vi "AB_Check_ConPane_For_Terminal_Type.vi"(8 "error in (no error)":errorcluster, 10 "Type Enum":T1, 11 "VI Path":path) -> (0 "error out":errorcluster, 3 "type found":bool)   [LabVIEW 2020]
uses:
  <vilib>/Utility/VariantDataType/Type.ctl
  <vilib>/Utility/VariantDataType/VariantType.lvlib
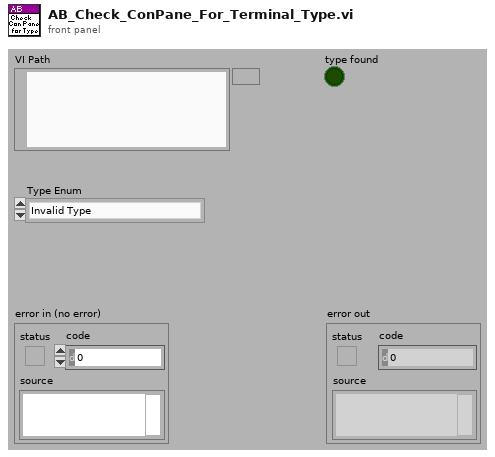
[diagram p1: front panel]
types:
  T1 = typedef "VariantType.lvlib/Type.ctl" = enum8{"Invalid Type", "Void", "I8", "I16", "I32", "I64", "U8", "U16", "U32", "U64", "Single Float", "Double Float", "Extended Float", "Single Complex", "Double Complex", "Extended Complex", "Enum U8", "Enum U16", "Enum U32", "Enum U64", "Single Float With Unit", "Double Float With Unit", "Extended Float With Unit", "Single Complex with Unit", "Double Complex with Unit", "Extended Complex with Unit", "Boolean", "String", "Path", "Picture", "Tag", "Array", "Cluster", "Variant", "LV Variant", "Waveform", "Timestamp", "Digital Waveform", "Digital Data", "ExpressData", "Refnum", "External Data", "VI", "Poly VI", "LabVIEW Class Instance", "Fixed Point"}
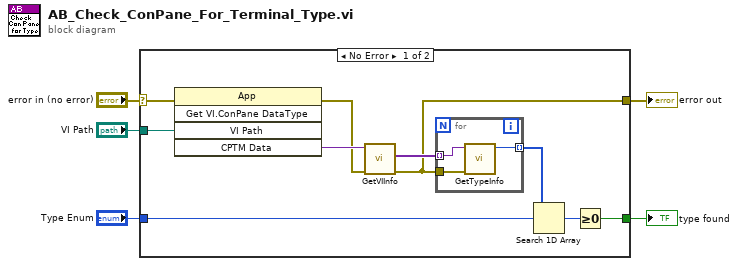
[diagram p0: block diagram]
diagram:
  n1 = case shown="No Error" "error in (no error)" {
    selector: "error in (no error)" -> [w14 w19]
    tunnel: "VI Path" -> [w15 _]
    tunnel: "Type Enum" -> [w9 _]
    tunnel: [w7 _] -> w2
    tunnel: [w6 w19] -> w1
    frame No Error {
      n2 = invoke class="App" method="Get VI.ConPane DataType"(error in=w14, "VI Path"=w15) -> (error out=w12:errorcluster, "CPTM Data"=w13:variant)  [unwired: 3 in, 3 out]
      n3 = call <vilib>:"GetVIInfo.vi"("error in (no error)"=w12, "Variant"=w13) -> ("error out"=w6:errorcluster, "VI Terminal Types"=w11:variant[])  [unwired: 5 in, 3 out]
      n4 = for {
        tunnel: w11 -> [w18] mode=indexing
        tunnel: [w17] -> w10 mode=indexing
        tunnel: w6 -> [w16]
        n5 = call <vilib>:"GetTypeInfo.vi"("error in (no error)"=w16, "Variant"=w18) -> ("Type Enum"=w17:T1)  [unwired: 5 in, 4 out]
      }
      n6 = Search 1D Array(1D array=w10, element=w9) -> (index of element=w8:i32)  [unwired: 1 in]
      n7 = Greater Or Equal To 0?(x=w8) -> (x >= 0?=w7:bool)
    }
    frame Error {
    }
  }
  "error out" <- w1
  "type found" <- w2
